vi "motorTest.vi"() -> ()   [LabVIEW 2017]
panel:
  in  "LCD":string
  in  "seven segment":i32
  in  "Motor B":dbl
  in  "Motor A":dbl
  in  "Stop Button":bool
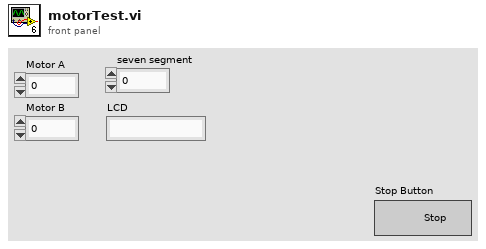
[diagram p1: front panel]
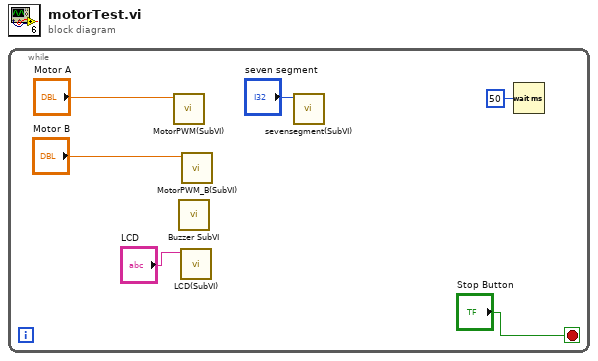
[diagram p0: block diagram]
diagram:
  n1 = while {
    stop <- "Stop Button" stop-if-true
    n2 = call "MotorPWM(SubVI).vi"("Duty Cycle (-100 to + 100)"="Motor A") -> ()  [unwired: 11 in]
    n3 = call "Buzzer SubVI.vi"() -> ()  [unwired: 12 in]
    n4 = call "LCD(SubVI).vi"("String"="LCD") -> ()  [unwired: 11 in]
    n5 = call "MotorPWM_B(SubVI).vi"("Duty Cycle (-100 to + 100)"="Motor B") -> ()  [unwired: 11 in]
    n6 = call "sevensegment(SubVI).vi"("Numeric"="seven segment") -> ()  [unwired: 11 in]
    n7 = Wait (ms)(milliseconds to wait=u32 50) -> ()  [unwired: 1 out]
  }
